vi "Periodic Tasks.vi"(8 "error in":errorcluster) -> ()   [LabVIEW 2015]
doc: "This VI runs in parallel to other tasks. It can contain as many user-defined periodic loops as you need. These can carry out PID or other sorts of timed response."
uses:
  <vilib>/Rock Robotics/SystemInterfaces/DIO/FPGA_DIOPWMChannel.ctl
  <vilib>/Rock Robotics/WPI/Utilities/WPI_GetSetVariantRefNum.vi
  <vilib>/Rock Robotics/WPI/MotorControl/WPI_MotorControlOpen TalonSRX.vi
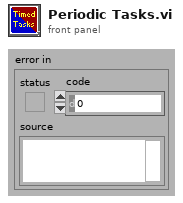
[diagram p1: front panel]
types:
  T1 = typedef "FPGA_DIOPWMChannel.ctl" = enum8{"PWM 0", "PWM 1", "PWM 2", "PWM 3", "PWM 4", "PWM 5", "PWM 6", "PWM 7", "PWM 8", "PWM 9", "PWM MXP 0", "PWM MXP 1", "PWM MXP 2", "PWM MXP 3", "PWM MXP 4", "PWM MXP 5", "PWM MXP 6", "PWM MXP 7", "PWM MXP 8", "PWM MXP 9", "Invalid"}
  T2 = typedef "WPI_JoystickDevRef.ctl" = cluster{"Device":T3}
  T3 = typedef "WPI_JoystickDeviceEnum.ctl" = enum16{"USB 0", "USB 1", "USB 2", "USB 3", "USB 4", "USB 5"}
  T4 = typedef "WPI_RobotDriveDevRef.ctl" = cluster{"DevStatus":errorcluster, "Motors[]":T5[], "Square Inputs":bool, "Max Output":dbl}
  T5 = typedef "WPI_MotorControlDeviceRef.ctl" = cluster{"DeviceStatus":errorcluster, "Type":T6, "PWM":cluster{"PWM Channel":T1, "DeadBand":T7}, "CAN":cluster{"Device Number":u8, "Control Mode":T8, "Semaphore":T9, "Max Vout":dbl, "TalonSRX Control Mode":T10}, "Invert":bool}
  T6 = typedef "WPI_MotorControlType.ctl" = enum16{"PWM", "CAN", "CANTalonSRX"}
  T7 = typedef "WPI_PWMDeadband.ctl" = cluster{"Name":string, "maxPositivePwm":i32, "minPositivePwm":i32, "centerPwm":i32, "maxNegativePwm":i32, "minNegativePwm":i32, "angularRange":u16}
  T8 = typedef "WPI_CANJaguar_ControlMode.ctl" = enum8{"Percent VBus", "Current", "Speed", "Position", "Voltage"}
  T9 = typedef "Semaphore RefNum" = refnum<k1>
  T10 = typedef "WPI_CANTalonSRX_APIControlMode.ctl" = enum8{"Percent VBus", "Speed", "Position", "Slave", "Unchanged / Invalid", "Voltage Compensation", "Current", "Motion Profile"}
  T11 = cluster{"JoystickDevRef":T2, "RobotDriveDevRef":T4}
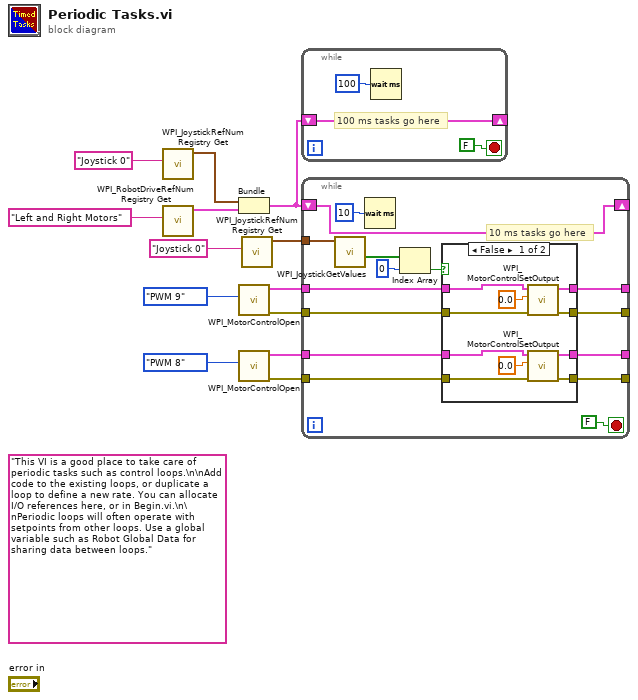
[diagram p0: block diagram]
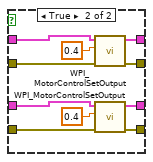
[diagram p2: hidden frame]
diagram:
  (unwired) "This VI is a good place to take care of periodic tasks such as control loops.\n\nAdd code to the existing loops, or duplicate a loop to define a new rate. You can allocate I/O references here, or in Begin.vi.\n\nPeriodic loops will often operate with setpoints from other loops. Use a global variable such as Robot Global Data for sharing data between loops."
  n1 = call <vilib>:"WPI_JoystickRefNum Registry Get.vi"("refnum name"="Joystick 0") -> ("JoystickDevRef"=w11:T2)  [unwired: 1 in, 9 out]
  n2 = call <vilib>:"WPI_RobotDriveRefNum Registry Get.vi"("refnum name"="Left and Right Motors") -> ("RobotDriveDevRef"=w10:T4)  [unwired: 1 in, 9 out]
  n3 = Bundle("JoystickDevRef"=w11, "RobotDriveDevRef"=w10) -> (w9:T11)  [unwired: 1 out]
  n4 = call-poly <vilib>:"WPI_MotorControlOpen.vi"("PWM Channel"=FPGA_DIOPWMChannel."PWM 9") -> ("error out"=w1:errorcluster, "MotorControlDeviceRef"=w3:T5)  [unwired: 9 in]
  n5 = call-poly <vilib>:"WPI_MotorControlOpen.vi"("PWM Channel"=FPGA_DIOPWMChannel."PWM 8") -> ("error out"=w2:errorcluster, "MotorControlDeviceRef"=w4:T5)  [unwired: 9 in]
  n6 = call <vilib>:"WPI_JoystickRefNum Registry Get.vi"("refnum name"="Joystick 0") -> ("JoystickDevRef"=w5:T2)  [unwired: 9 in, 1 out]
  n7 = while {
    shift-right: [w14] -> _
    shift-left: w9 -> [w14]
    stop <- FALSE stop-if-true
    # "100 ms tasks go here"
    n8 = Wait (ms)(milliseconds to wait=u32 100) -> ()  [unwired: 1 out]
  }
  n9 = while {
    shift-right: [w29] -> _
    shift-left: w9 -> [w29]
    tunnel: w5 -> [w28]
    tunnel: w4 -> [w25]
    tunnel: w3 -> [w24]
    tunnel: w2 -> [w23]
    tunnel: w1 -> [w22]
    tunnel: [w21] -> _
    tunnel: [w20] -> _
    tunnel: [w19] -> _
    tunnel: [w18] -> _
    stop <- FALSE stop-if-true
    # "10 ms tasks go here"
    n10 = call <vilib>:"WPI_JoystickGetValues.vi"("JoystickDevRef"=w28) -> ("Buttons"=w27:bool[])  [unwired: 6 in, 4 out]
    n11 = Wait (ms)(milliseconds to wait=u32 10) -> ()  [unwired: 1 out]
    n12 = Index Array(array=w27, index=0) -> (element=w26:bool)
    n13 = case shown="False" w26 {
      tunnel: w25 -> [w33 w51]
      tunnel: w24 -> [w40 w50]
      tunnel: w23 -> [w32 w47]
      tunnel: w22 -> [w39 w46]
      tunnel: [w35 w45] -> w21
      tunnel: [w36 w44] -> w20
      tunnel: [w37 w43] -> w19
      tunnel: [w38 w42] -> w18
      frame False {
        n14 = call <vilib>:"WPI_MotorControlSetOutput.vi"("error in (no error)"=w39, "Output"=0.0, "MotorControlDevRef"=w40) -> ("error out"=w38:errorcluster, "MotorControlDevRef"=w37:T5)  [unwired: 6 in, 1 out]
        n15 = call <vilib>:"WPI_MotorControlSetOutput.vi"("error in (no error)"=w32, "Output"=0.0, "MotorControlDevRef"=w33) -> ("error out"=w36:errorcluster, "MotorControlDevRef"=w35:T5)  [unwired: 6 in, 1 out]
      }
      frame True {
        n16 = call <vilib>:"WPI_MotorControlSetOutput.vi"("error in (no error)"=w46, "Output"=0.4, "MotorControlDevRef"=w50) -> ("error out"=w42:errorcluster, "MotorControlDevRef"=w43:T5)  [unwired: 6 in, 1 out]
        n17 = call <vilib>:"WPI_MotorControlSetOutput.vi"("error in (no error)"=w47, "Output"=0.4, "MotorControlDevRef"=w51) -> ("error out"=w44:errorcluster, "MotorControlDevRef"=w45:T5)  [unwired: 6 in, 1 out]
      }
    }
  }
